vi "OCR Player Money.vi"(7 "error in":errorcluster) -> (17 "String (Player10 Money)":string, 18 "String (Player 9 Money)":string, 19 "String (Player8 Money)":string, 20 "String (Player1 Money)":string, 21 "String (Player2 Money)":string, 22 "String (Player3 Money)":string, 23 "String (Player4 Money)":string, 24 "String (Player5 Money)":string, 25 "String (Player6 Money)":string, 26 "String (Player7 Money)":string, 27 "error out":errorcluster)   [LabVIEW 2015]
uses:
  <vilib>/vision/NI_Vision_Development_Module.lvlib
panel:
  out "Player Money":string[](array[string])
  in  "SS Path":path=path "c:/PokerSS/SS.png"
  out "Image Out":T1(plugin-control)
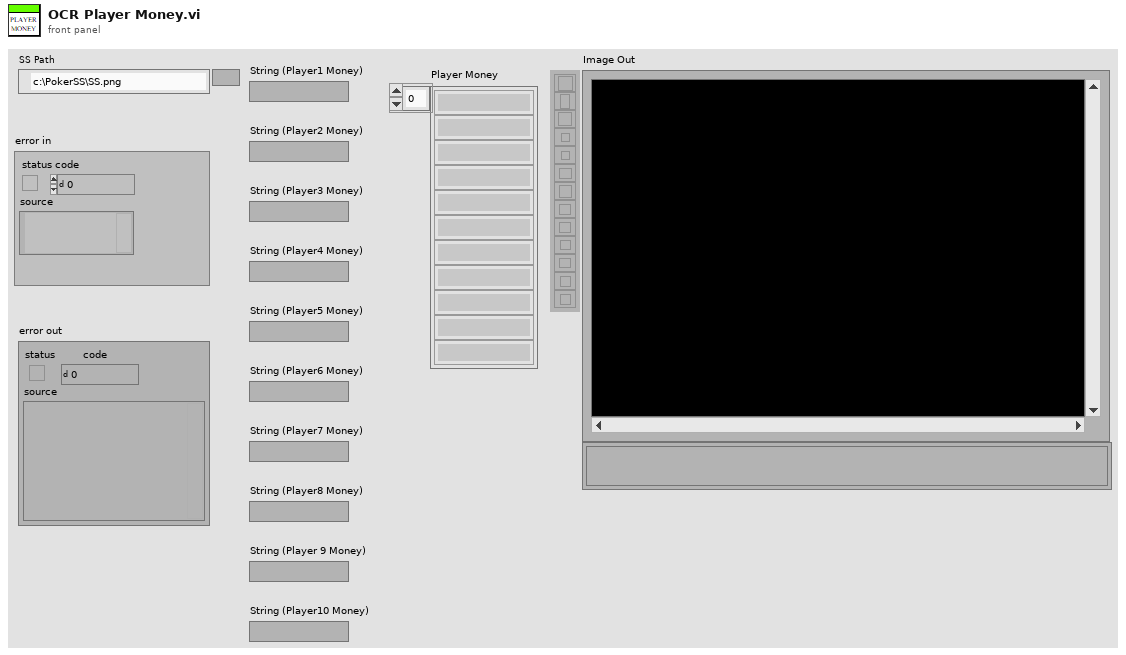
[diagram p1: front panel]
types:
  T1 = typedef "IMAQ Image.ctl" = refnum<image>
  T2 = cluster{"Threshold Data":cluster{"Method":enum16{"Fixed Range", "Uniform", "Linear", "Non Linear", "Local", "Color"}, "Looking for":u32, "Color Mode":u32, "Kernel Size":cluster{"Width":i32, "Height":i32}, "Ranges":cluster{"Min":i32, "Max":i32}[]}, "Reject Border":bool, "Number Of Erosions":i32, "Size & Spacing":cluster{"Segment Algorithm":u16, "Min Bounding Rect Width":i32, "Max Bounding Rect Width":i32, "Min Bounding Rect Height":i32, "Max Bounding Rect Height":i32, "Min Character Size":i32, "Max Character Size":i32, "Min Char Spacing":i32, "Max Horiz Element Spacing":i32, "Max Vert Element Spacing":i32, "Max Space Distance":i32}, "Read Options":cluster{"Read Strategy":i32, "Read Resolution":i32, "Scale Dependant":bool, "Aspect Ratio":i32, "Acceptance Level":i32, "Substitution Character":string, "MultiLine":bool}, "Valid Characters":cluster{"Pre-defined characters":i32, "User-defined characters":string}[], "Use Text Pattern":bool, "Orientation":u32, "# Lines Expected":u32, "Number of Blocks":i32}
  T3 = cluster{"Global Rectangle":i32[], "Contours":cluster{"ID":enum32{"External", "Internal"}, "Type":u32, "Coordinates":i32[]}[]}
  T4 = typedef "Image Type" = u32
  T5 = typedef "IMAQ OCR Session.ctl" = refnum<k1>
diagram:
  (unwired) path "C:/Users/Bob Dabalina/Documents/Labview/OCR Practice/Views Numbers.abc" ("File Path")
  w26 = u32 0 items=["Grayscale", "Binary", "Gradient", "Rainbow", "Temperature", "User Defined", "Binary 16 Bit", "Gradient 16 Bit", "Rainbow 16 Bit", "Temperature 16 Bit", "User Defined 16 Bit"] ("Palette Type")
  w35 = T2 {"Threshold Data"={"Method"=enum."Uniform", "Looking for"=1, "Color Mode"=0, "Kernel Size"={"Width"=32, "Height"=32}, "Ranges"=[{"Min"=1, "Max"=255}]}, "Reject Border"=TRUE, "Number Of Erosions"=0, "Size & Spacing"={"Segment Algorithm"=0, "Min Bounding Rect Width"=2, "Max Bounding Rect Width"=8, "Min Bounding Rect Height"=2, "Max Bounding Rect Height"=65536, "Min Character Size"=4, "Max Character Size"=5555, "Min Char Spacing"=1, "Max Horiz Element Spacing"=1, "Max Vert Element Spacing"=0, "Max Space Distance"=65536}, "Read Options"={"Read Strategy"=1, "Read Resolution"=2, "Scale Dependant"=FALSE, "Aspect Ratio"=400, "Acceptance Level"=700, "Substitution Character"="?", "MultiLine"=FALSE}, "Valid Characters"=[], "Use Text Pattern"=FALSE, "Orientation"=0, "# Lines Expected"=0, "Number of Blocks"=4}  # Parameters
  w36 = T3 {"Global Rectangle"=[720, 494, 833, 510], "Contours"=[{"ID"=enum."External", "Type"=3, "Coordinates"=[720, 494, 833, 510]}]}  # ROI Descriptor
  w44 = T2 {"Threshold Data"={"Method"=enum."Uniform", "Looking for"=1, "Color Mode"=0, "Kernel Size"={"Width"=32, "Height"=32}, "Ranges"=[{"Min"=1, "Max"=255}]}, "Reject Border"=TRUE, "Number Of Erosions"=0, "Size & Spacing"={"Segment Algorithm"=0, "Min Bounding Rect Width"=2, "Max Bounding Rect Width"=8, "Min Bounding Rect Height"=2, "Max Bounding Rect Height"=65536, "Min Character Size"=4, "Max Character Size"=5555, "Min Char Spacing"=1, "Max Horiz Element Spacing"=1, "Max Vert Element Spacing"=0, "Max Space Distance"=65536}, "Read Options"={"Read Strategy"=1, "Read Resolution"=2, "Scale Dependant"=FALSE, "Aspect Ratio"=400, "Acceptance Level"=700, "Substitution Character"="?", "MultiLine"=FALSE}, "Valid Characters"=[], "Use Text Pattern"=FALSE, "Orientation"=0, "# Lines Expected"=0, "Number of Blocks"=4}  # Parameters
  w45 = T3 {"Global Rectangle"=[523, 533, 645, 550], "Contours"=[{"ID"=enum."External", "Type"=3, "Coordinates"=[523, 533, 645, 550]}]}  # ROI Descriptor
  w53 = T2 {"Threshold Data"={"Method"=enum."Uniform", "Looking for"=1, "Color Mode"=0, "Kernel Size"={"Width"=32, "Height"=32}, "Ranges"=[{"Min"=1, "Max"=255}]}, "Reject Border"=TRUE, "Number Of Erosions"=0, "Size & Spacing"={"Segment Algorithm"=0, "Min Bounding Rect Width"=2, "Max Bounding Rect Width"=8, "Min Bounding Rect Height"=2, "Max Bounding Rect Height"=65536, "Min Character Size"=4, "Max Character Size"=5555, "Min Char Spacing"=1, "Max Horiz Element Spacing"=1, "Max Vert Element Spacing"=0, "Max Space Distance"=65536}, "Read Options"={"Read Strategy"=1, "Read Resolution"=2, "Scale Dependant"=FALSE, "Aspect Ratio"=400, "Acceptance Level"=700, "Substitution Character"="?", "MultiLine"=FALSE}, "Valid Characters"=[], "Use Text Pattern"=FALSE, "Orientation"=0, "# Lines Expected"=0, "Number of Blocks"=4}  # Parameters
  w54 = T3 {"Global Rectangle"=[386, 689, 502, 706], "Contours"=[{"ID"=enum."External", "Type"=3, "Coordinates"=[386, 689, 502, 706]}]}  # ROI Descriptor
  w62 = T2 {"Threshold Data"={"Method"=enum."Uniform", "Looking for"=1, "Color Mode"=0, "Kernel Size"={"Width"=32, "Height"=32}, "Ranges"=[{"Min"=1, "Max"=255}]}, "Reject Border"=TRUE, "Number Of Erosions"=0, "Size & Spacing"={"Segment Algorithm"=0, "Min Bounding Rect Width"=2, "Max Bounding Rect Width"=8, "Min Bounding Rect Height"=2, "Max Bounding Rect Height"=65536, "Min Character Size"=4, "Max Character Size"=5555, "Min Char Spacing"=1, "Max Horiz Element Spacing"=1, "Max Vert Element Spacing"=0, "Max Space Distance"=65536}, "Read Options"={"Read Strategy"=1, "Read Resolution"=2, "Scale Dependant"=FALSE, "Aspect Ratio"=400, "Acceptance Level"=700, "Substitution Character"="?", "MultiLine"=FALSE}, "Valid Characters"=[], "Use Text Pattern"=FALSE, "Orientation"=0, "# Lines Expected"=0, "Number of Blocks"=4}  # Parameters
  w63 = T3 {"Global Rectangle"=[543, 836, 661, 852], "Contours"=[{"ID"=enum."External", "Type"=3, "Coordinates"=[543, 836, 661, 852]}]}  # ROI Descriptor
  w71 = T2 {"Threshold Data"={"Method"=enum."Uniform", "Looking for"=1, "Color Mode"=0, "Kernel Size"={"Width"=32, "Height"=32}, "Ranges"=[{"Min"=1, "Max"=255}]}, "Reject Border"=TRUE, "Number Of Erosions"=0, "Size & Spacing"={"Segment Algorithm"=0, "Min Bounding Rect Width"=2, "Max Bounding Rect Width"=8, "Min Bounding Rect Height"=2, "Max Bounding Rect Height"=65536, "Min Character Size"=4, "Max Character Size"=5555, "Min Char Spacing"=1, "Max Horiz Element Spacing"=1, "Max Vert Element Spacing"=0, "Max Space Distance"=65536}, "Read Options"={"Read Strategy"=1, "Read Resolution"=2, "Scale Dependant"=FALSE, "Aspect Ratio"=400, "Acceptance Level"=700, "Substitution Character"="?", "MultiLine"=FALSE}, "Valid Characters"=[], "Use Text Pattern"=FALSE, "Orientation"=0, "# Lines Expected"=0, "Number of Blocks"=4}  # Parameters
  w72 = T3 {"Global Rectangle"=[757, 870, 877, 885], "Contours"=[{"ID"=enum."External", "Type"=3, "Coordinates"=[757, 870, 877, 885]}]}  # ROI Descriptor
  w80 = T2 {"Threshold Data"={"Method"=enum."Uniform", "Looking for"=1, "Color Mode"=0, "Kernel Size"={"Width"=32, "Height"=32}, "Ranges"=[{"Min"=1, "Max"=255}]}, "Reject Border"=TRUE, "Number Of Erosions"=0, "Size & Spacing"={"Segment Algorithm"=0, "Min Bounding Rect Width"=2, "Max Bounding Rect Width"=8, "Min Bounding Rect Height"=2, "Max Bounding Rect Height"=65536, "Min Character Size"=4, "Max Character Size"=5555, "Min Char Spacing"=1, "Max Horiz Element Spacing"=1, "Max Vert Element Spacing"=0, "Max Space Distance"=65536}, "Read Options"={"Read Strategy"=1, "Read Resolution"=2, "Scale Dependant"=FALSE, "Aspect Ratio"=400, "Acceptance Level"=700, "Substitution Character"="?", "MultiLine"=FALSE}, "Valid Characters"=[], "Use Text Pattern"=FALSE, "Orientation"=0, "# Lines Expected"=0, "Number of Blocks"=4}  # Parameters
  w81 = T3 {"Global Rectangle"=[1029, 868, 1143, 884], "Contours"=[{"ID"=enum."External", "Type"=3, "Coordinates"=[1029, 868, 1143, 884]}]}  # ROI Descriptor
  w89 = T2 {"Threshold Data"={"Method"=enum."Uniform", "Looking for"=1, "Color Mode"=0, "Kernel Size"={"Width"=32, "Height"=32}, "Ranges"=[{"Min"=1, "Max"=255}]}, "Reject Border"=TRUE, "Number Of Erosions"=0, "Size & Spacing"={"Segment Algorithm"=0, "Min Bounding Rect Width"=2, "Max Bounding Rect Width"=8, "Min Bounding Rect Height"=2, "Max Bounding Rect Height"=65536, "Min Character Size"=4, "Max Character Size"=5555, "Min Char Spacing"=1, "Max Horiz Element Spacing"=1, "Max Vert Element Spacing"=0, "Max Space Distance"=65536}, "Read Options"={"Read Strategy"=1, "Read Resolution"=2, "Scale Dependant"=FALSE, "Aspect Ratio"=400, "Acceptance Level"=700, "Substitution Character"="?", "MultiLine"=FALSE}, "Valid Characters"=[], "Use Text Pattern"=FALSE, "Orientation"=0, "# Lines Expected"=0, "Number of Blocks"=4}  # Parameters
  w90 = T3 {"Global Rectangle"=[1264, 838, 1374, 853], "Contours"=[{"ID"=enum."External", "Type"=3, "Coordinates"=[1264, 838, 1374, 853]}]}  # ROI Descriptor
  w98 = T2 {"Threshold Data"={"Method"=enum."Uniform", "Looking for"=1, "Color Mode"=0, "Kernel Size"={"Width"=32, "Height"=32}, "Ranges"=[{"Min"=1, "Max"=255}]}, "Reject Border"=TRUE, "Number Of Erosions"=0, "Size & Spacing"={"Segment Algorithm"=0, "Min Bounding Rect Width"=2, "Max Bounding Rect Width"=8, "Min Bounding Rect Height"=2, "Max Bounding Rect Height"=65536, "Min Character Size"=4, "Max Character Size"=5555, "Min Char Spacing"=1, "Max Horiz Element Spacing"=1, "Max Vert Element Spacing"=0, "Max Space Distance"=65536}, "Read Options"={"Read Strategy"=1, "Read Resolution"=2, "Scale Dependant"=FALSE, "Aspect Ratio"=400, "Acceptance Level"=700, "Substitution Character"="?", "MultiLine"=FALSE}, "Valid Characters"=[], "Use Text Pattern"=FALSE, "Orientation"=0, "# Lines Expected"=0, "Number of Blocks"=4}  # Parameters
  w99 = T3 {"Global Rectangle"=[1385, 697, 1502, 712], "Contours"=[{"ID"=enum."External", "Type"=3, "Coordinates"=[1385, 697, 1502, 712]}]}  # ROI Descriptor
  w107 = T2 {"Threshold Data"={"Method"=enum."Uniform", "Looking for"=1, "Color Mode"=0, "Kernel Size"={"Width"=32, "Height"=32}, "Ranges"=[{"Min"=1, "Max"=255}]}, "Reject Border"=TRUE, "Number Of Erosions"=0, "Size & Spacing"={"Segment Algorithm"=0, "Min Bounding Rect Width"=2, "Max Bounding Rect Width"=8, "Min Bounding Rect Height"=2, "Max Bounding Rect Height"=65536, "Min Character Size"=4, "Max Character Size"=5555, "Min Char Spacing"=1, "Max Horiz Element Spacing"=1, "Max Vert Element Spacing"=0, "Max Space Distance"=65536}, "Read Options"={"Read Strategy"=1, "Read Resolution"=2, "Scale Dependant"=FALSE, "Aspect Ratio"=400, "Acceptance Level"=700, "Substitution Character"="?", "MultiLine"=FALSE}, "Valid Characters"=[], "Use Text Pattern"=FALSE, "Orientation"=0, "# Lines Expected"=0, "Number of Blocks"=4}  # Parameters
  w108 = T3 {"Global Rectangle"=[1068, 495, 1179, 512], "Contours"=[{"ID"=enum."External", "Type"=3, "Coordinates"=[1068, 495, 1179, 512]}]}  # ROI Descriptor
  w116 = T2 {"Threshold Data"={"Method"=enum."Uniform", "Looking for"=1, "Color Mode"=0, "Kernel Size"={"Width"=32, "Height"=32}, "Ranges"=[{"Min"=1, "Max"=255}]}, "Reject Border"=TRUE, "Number Of Erosions"=0, "Size & Spacing"={"Segment Algorithm"=0, "Min Bounding Rect Width"=2, "Max Bounding Rect Width"=8, "Min Bounding Rect Height"=2, "Max Bounding Rect Height"=65536, "Min Character Size"=4, "Max Character Size"=5555, "Min Char Spacing"=1, "Max Horiz Element Spacing"=1, "Max Vert Element Spacing"=0, "Max Space Distance"=65536}, "Read Options"={"Read Strategy"=1, "Read Resolution"=2, "Scale Dependant"=FALSE, "Aspect Ratio"=400, "Acceptance Level"=700, "Substitution Character"="?", "MultiLine"=FALSE}, "Valid Characters"=[], "Use Text Pattern"=FALSE, "Orientation"=0, "# Lines Expected"=0, "Number of Blocks"=4}  # Parameters
  w117 = T3 {"Global Rectangle"=[1068, 495, 1179, 512], "Contours"=[{"ID"=enum."External", "Type"=3, "Coordinates"=[1068, 495, 1179, 512]}]}  # ROI Descriptor
  w120 = 1 items=["Red", "Green", "Blue", "Hue", "Saturation", "Luminance", "Value", "Intensity"] ("Color Plane")
  w121 = T4 4 items=["Grayscale (U8)", "Grayscale (I16)", "Grayscale (SGL)", "Complex (CSG)", "RGB (U32)", "HSL (U32)", "RGB (U64)", "Grayscale (U16)"] ("Image Type")
  # "Create player money array"
  n1 = Call Chain() -> (call chain=w123:string[])
  n2 = Index Array(array=w123) -> (element=w122:string)  [unwired: 1 in]
  n3 = call "IMAQ Create"("Image Name"=w122, "Image Type"=w121, "error in (no error)"="error in") -> ("New Image"=w126:T1, "error out"=w125:errorcluster)  [unwired: 1 in, 1 out]
  n4 = call "IMAQ ReadFile"("File Path"="SS Path", "error in (no error)"=w125, "Image"=w126) -> ("error out"=w127:errorcluster, "Image Out"=w119:T1)  [unwired: 2 in, 5 out]
  n5 = call "IMAQ ExtractSingleColorPlane"("Color Plane"=w120, "error in (no error)"=w127, "Image Src"=w119) -> ("error out"=w118:errorcluster, "Image Dst Out"=w27:T1)  [unwired: 1 in, 6 out]
  "Image Out" <- w27
  n6 = while "Create an OCR session and read the character set file.\nSet paramaters from Vision Assistant Step." {
    shift-right: [w132] -> w114
    shift-left: _ -> [w131]
    tunnel: w118 -> [w134]
    tunnel: w116 -> [w130]
    tunnel: path "C:/Users/Bob Dabalina/Documents/Labview/OCR Practice/Views Numbers.abc" ("File Path") -> [w129]
    tunnel: [w128] -> w115
    stop <- FALSE continue-if-true
    n7 = First Call?() -> (First Call?: T/F=w133:bool)
    n8 = case shown="True" w133 {
      tunnel: w129 -> [_ w141]
      tunnel: w134 -> [w136 w145]
      tunnel: [w137 w143] -> w132
      tunnel: [w136 w142] -> w128
      tunnel: w130 -> [_ w138]
      tunnel: w131 -> [w137 _]
      frame False {
      }
      frame True {
        w146 = 0 items=["Read All", "Read Character Set Only", "Read Properties Only"] ("Read Options")
        n9 = call <vilib>:"IVA Get Alternate Path.vi"("Path In"=w141) -> ("Path Out"=w140:path)  [unwired: 10 out]
        n10 = call "IMAQ OCR Create Session"("error in (no error)"=w145) -> ("error out"=w147:errorcluster, "IMAQ OCR Session"=w148:T5)  [unwired: 9 out]
        n11 = call "IMAQ OCR Read Character Set File"("File Path"=w140, "error in (no error)"=w147, "Read Options"=w146, "IMAQ OCR Session"=w148) -> ("error out"=w144:errorcluster, "IMAQ OCR Session (dup)"=w139:T5)  [unwired: 1 in, 5 out]
        n12 = call <vilib>:"IVA OCR - Set Parameters 2.vi"("error in (no error)"=w144, "Parameters"=w138, "IMAQ OCR Session"=w139) -> ("error out"=w142:errorcluster, "IMAQ OCR Session Out"=w143:T5)  [unwired: 7 in]
      }
    }
  }
  n13 = Unbundle By Name(w116) -> ("# Lines Expected"=w112:u32, "Orientation"=w113:u32)
  n14 = call "IMAQ OCR Read Text 4"("IMAQ OCR Session"=w114, "ROI Descriptor"=w117, "Image"=w27, "Number of Lines Requested"=w112, "error in (no error)"=w115, "Orientation"=w113) -> ("Read String"=w20:string, "error out"=w111:errorcluster)  [unwired: 8 out]
  "String (Player1 Money)" <- w20
  n15 = call <vilib>:"IVA Clear Coordsys Errors.vi"("error in (no error)"=w111) -> ("error out"=w110:errorcluster)  [unwired: 10 in]
  n16 = Initialize Array("") -> (w22:string[])  [unwired: 1 in]
  n17 = Insert Into Array(array=w22, index=0, new element=w20) -> (w19:string[])
  n18 = while "Create an OCR session and read the character set file.\nSet paramaters from Vision Assistant Step." {
    shift-right: [w153] -> w105
    shift-left: _ -> [w152]
    tunnel: w110 -> [w155]
    tunnel: w107 -> [w151]
    tunnel: path "C:/Users/Bob Dabalina/Documents/Labview/OCR Practice/Views Numbers.abc" ("File Path") -> [w150]
    tunnel: [w149] -> w106
    stop <- FALSE continue-if-true
    n19 = First Call?() -> (First Call?: T/F=w154:bool)
    n20 = case shown="True" w154 {
      tunnel: w150 -> [_ w162]
      tunnel: w155 -> [w157 w166]
      tunnel: [w158 w164] -> w153
      tunnel: [w157 w163] -> w149
      tunnel: w151 -> [_ w159]
      tunnel: w152 -> [w158 _]
      frame False {
      }
      frame True {
        w167 = 0 items=["Read All", "Read Character Set Only", "Read Properties Only"] ("Read Options")
        n21 = call <vilib>:"IVA Get Alternate Path.vi"("Path In"=w162) -> ("Path Out"=w161:path)  [unwired: 10 out]
        n22 = call "IMAQ OCR Create Session"("error in (no error)"=w166) -> ("error out"=w168:errorcluster, "IMAQ OCR Session"=w169:T5)  [unwired: 9 out]
        n23 = call "IMAQ OCR Read Character Set File"("File Path"=w161, "error in (no error)"=w168, "Read Options"=w167, "IMAQ OCR Session"=w169) -> ("error out"=w165:errorcluster, "IMAQ OCR Session (dup)"=w160:T5)  [unwired: 1 in, 5 out]
        n24 = call <vilib>:"IVA OCR - Set Parameters 2.vi"("error in (no error)"=w165, "Parameters"=w159, "IMAQ OCR Session"=w160) -> ("error out"=w163:errorcluster, "IMAQ OCR Session Out"=w164:T5)  [unwired: 7 in]
      }
    }
  }
  n25 = Unbundle By Name(w107) -> ("# Lines Expected"=w103:u32, "Orientation"=w104:u32)
  n26 = call "IMAQ OCR Read Text 4"("IMAQ OCR Session"=w105, "ROI Descriptor"=w108, "Image"=w27, "Number of Lines Requested"=w103, "error in (no error)"=w106, "Orientation"=w104) -> ("Read String"=w18:string, "error out"=w102:errorcluster)  [unwired: 8 out]
  "String (Player2 Money)" <- w18
  n27 = call <vilib>:"IVA Clear Coordsys Errors.vi"("error in (no error)"=w102) -> ("error out"=w101:errorcluster)  [unwired: 10 in]
  n28 = Build Array (concatenate)(w19, w18) -> (w17:string[])
  n29 = while "Create an OCR session and read the character set file.\nSet paramaters from Vision Assistant Step." {
    shift-right: [w174] -> w96
    shift-left: _ -> [w173]
    tunnel: w101 -> [w176]
    tunnel: w98 -> [w172]
    tunnel: path "C:/Users/Bob Dabalina/Documents/Labview/OCR Practice/Views Numbers.abc" ("File Path") -> [w171]
    tunnel: [w170] -> w97
    stop <- FALSE continue-if-true
    n30 = First Call?() -> (First Call?: T/F=w175:bool)
    n31 = case shown="True" w175 {
      tunnel: w171 -> [_ w183]
      tunnel: w176 -> [w178 w187]
      tunnel: [w179 w185] -> w174
      tunnel: [w178 w184] -> w170
      tunnel: w172 -> [_ w180]
      tunnel: w173 -> [w179 _]
      frame False {
      }
      frame True {
        w188 = 0 items=["Read All", "Read Character Set Only", "Read Properties Only"] ("Read Options")
        n32 = call <vilib>:"IVA Get Alternate Path.vi"("Path In"=w183) -> ("Path Out"=w182:path)  [unwired: 10 out]
        n33 = call "IMAQ OCR Create Session"("error in (no error)"=w187) -> ("error out"=w189:errorcluster, "IMAQ OCR Session"=w190:T5)  [unwired: 9 out]
        n34 = call "IMAQ OCR Read Character Set File"("File Path"=w182, "error in (no error)"=w189, "Read Options"=w188, "IMAQ OCR Session"=w190) -> ("error out"=w186:errorcluster, "IMAQ OCR Session (dup)"=w181:T5)  [unwired: 1 in, 5 out]
        n35 = call <vilib>:"IVA OCR - Set Parameters 2.vi"("error in (no error)"=w186, "Parameters"=w180, "IMAQ OCR Session"=w181) -> ("error out"=w184:errorcluster, "IMAQ OCR Session Out"=w185:T5)  [unwired: 7 in]
      }
    }
  }
  n36 = Unbundle By Name(w98) -> ("# Lines Expected"=w94:u32, "Orientation"=w95:u32)
  n37 = call "IMAQ OCR Read Text 4"("IMAQ OCR Session"=w96, "ROI Descriptor"=w99, "Image"=w27, "Number of Lines Requested"=w94, "error in (no error)"=w97, "Orientation"=w95) -> ("Read String"=w16:string, "error out"=w93:errorcluster)  [unwired: 8 out]
  "String (Player3 Money)" <- w16
  n38 = call <vilib>:"IVA Clear Coordsys Errors.vi"("error in (no error)"=w93) -> ("error out"=w92:errorcluster)  [unwired: 10 in]
  n39 = Build Array (concatenate)(w17, w16) -> (w15:string[])
  n40 = while "Create an OCR session and read the character set file.\nSet paramaters from Vision Assistant Step." {
    shift-right: [w195] -> w87
    shift-left: _ -> [w194]
    tunnel: w92 -> [w197]
    tunnel: w89 -> [w193]
    tunnel: path "C:/Users/Bob Dabalina/Documents/Labview/OCR Practice/Views Numbers.abc" ("File Path") -> [w192]
    tunnel: [w191] -> w88
    stop <- FALSE continue-if-true
    n41 = First Call?() -> (First Call?: T/F=w196:bool)
    n42 = case shown="True" w196 {
      tunnel: w192 -> [_ w204]
      tunnel: w197 -> [w199 w208]
      tunnel: [w200 w206] -> w195
      tunnel: [w199 w205] -> w191
      tunnel: w193 -> [_ w201]
      tunnel: w194 -> [w200 _]
      frame False {
      }
      frame True {
        w209 = 0 items=["Read All", "Read Character Set Only", "Read Properties Only"] ("Read Options")
        n43 = call <vilib>:"IVA Get Alternate Path.vi"("Path In"=w204) -> ("Path Out"=w203:path)  [unwired: 10 out]
        n44 = call "IMAQ OCR Create Session"("error in (no error)"=w208) -> ("error out"=w210:errorcluster, "IMAQ OCR Session"=w211:T5)  [unwired: 9 out]
        n45 = call "IMAQ OCR Read Character Set File"("File Path"=w203, "error in (no error)"=w210, "Read Options"=w209, "IMAQ OCR Session"=w211) -> ("error out"=w207:errorcluster, "IMAQ OCR Session (dup)"=w202:T5)  [unwired: 1 in, 5 out]
        n46 = call <vilib>:"IVA OCR - Set Parameters 2.vi"("error in (no error)"=w207, "Parameters"=w201, "IMAQ OCR Session"=w202) -> ("error out"=w205:errorcluster, "IMAQ OCR Session Out"=w206:T5)  [unwired: 7 in]
      }
    }
  }
  n47 = Unbundle By Name(w89) -> ("# Lines Expected"=w85:u32, "Orientation"=w86:u32)
  n48 = call "IMAQ OCR Read Text 4"("IMAQ OCR Session"=w87, "ROI Descriptor"=w90, "Image"=w27, "Number of Lines Requested"=w85, "error in (no error)"=w88, "Orientation"=w86) -> ("Read String"=w14:string, "error out"=w84:errorcluster)  [unwired: 8 out]
  "String (Player4 Money)" <- w14
  n49 = call <vilib>:"IVA Clear Coordsys Errors.vi"("error in (no error)"=w84) -> ("error out"=w83:errorcluster)  [unwired: 10 in]
  n50 = Build Array (concatenate)(w15, w14) -> (w13:string[])
  n51 = while "Create an OCR session and read the character set file.\nSet paramaters from Vision Assistant Step." {
    shift-right: [w216] -> w78
    shift-left: _ -> [w215]
    tunnel: w83 -> [w218]
    tunnel: w80 -> [w214]
    tunnel: path "C:/Users/Bob Dabalina/Documents/Labview/OCR Practice/Views Numbers.abc" ("File Path") -> [w213]
    tunnel: [w212] -> w79
    stop <- FALSE continue-if-true
    n52 = First Call?() -> (First Call?: T/F=w217:bool)
    n53 = case shown="True" w217 {
      tunnel: w213 -> [_ w225]
      tunnel: w218 -> [w220 w229]
      tunnel: [w221 w227] -> w216
      tunnel: [w220 w226] -> w212
      tunnel: w214 -> [_ w222]
      tunnel: w215 -> [w221 _]
      frame False {
      }
      frame True {
        w230 = 0 items=["Read All", "Read Character Set Only", "Read Properties Only"] ("Read Options")
        n54 = call <vilib>:"IVA Get Alternate Path.vi"("Path In"=w225) -> ("Path Out"=w224:path)  [unwired: 10 out]
        n55 = call "IMAQ OCR Create Session"("error in (no error)"=w229) -> ("error out"=w231:errorcluster, "IMAQ OCR Session"=w232:T5)  [unwired: 9 out]
        n56 = call "IMAQ OCR Read Character Set File"("File Path"=w224, "error in (no error)"=w231, "Read Options"=w230, "IMAQ OCR Session"=w232) -> ("error out"=w228:errorcluster, "IMAQ OCR Session (dup)"=w223:T5)  [unwired: 1 in, 5 out]
        n57 = call <vilib>:"IVA OCR - Set Parameters 2.vi"("error in (no error)"=w228, "Parameters"=w222, "IMAQ OCR Session"=w223) -> ("error out"=w226:errorcluster, "IMAQ OCR Session Out"=w227:T5)  [unwired: 7 in]
      }
    }
  }
  n58 = Unbundle By Name(w80) -> ("# Lines Expected"=w76:u32, "Orientation"=w77:u32)
  n59 = call "IMAQ OCR Read Text 4"("IMAQ OCR Session"=w78, "ROI Descriptor"=w81, "Image"=w27, "Number of Lines Requested"=w76, "error in (no error)"=w79, "Orientation"=w77) -> ("Read String"=w12:string, "error out"=w75:errorcluster)  [unwired: 8 out]
  "String (Player5 Money)" <- w12
  n60 = call <vilib>:"IVA Clear Coordsys Errors.vi"("error in (no error)"=w75) -> ("error out"=w74:errorcluster)  [unwired: 10 in]
  n61 = Build Array (concatenate)(w13, w12) -> (w11:string[])
  n62 = while "Create an OCR session and read the character set file.\nSet paramaters from Vision Assistant Step." {
    shift-right: [w237] -> w69
    shift-left: _ -> [w236]
    tunnel: w74 -> [w239]
    tunnel: w71 -> [w235]
    tunnel: path "C:/Users/Bob Dabalina/Documents/Labview/OCR Practice/Views Numbers.abc" ("File Path") -> [w234]
    tunnel: [w233] -> w70
    stop <- FALSE continue-if-true
    n63 = First Call?() -> (First Call?: T/F=w238:bool)
    n64 = case shown="True" w238 {
      tunnel: w234 -> [_ w246]
      tunnel: w239 -> [w241 w250]
      tunnel: [w242 w248] -> w237
      tunnel: [w241 w247] -> w233
      tunnel: w235 -> [_ w243]
      tunnel: w236 -> [w242 _]
      frame False {
      }
      frame True {
        w251 = 0 items=["Read All", "Read Character Set Only", "Read Properties Only"] ("Read Options")
        n65 = call <vilib>:"IVA Get Alternate Path.vi"("Path In"=w246) -> ("Path Out"=w245:path)  [unwired: 10 out]
        n66 = call "IMAQ OCR Create Session"("error in (no error)"=w250) -> ("error out"=w252:errorcluster, "IMAQ OCR Session"=w253:T5)  [unwired: 9 out]
        n67 = call "IMAQ OCR Read Character Set File"("File Path"=w245, "error in (no error)"=w252, "Read Options"=w251, "IMAQ OCR Session"=w253) -> ("error out"=w249:errorcluster, "IMAQ OCR Session (dup)"=w244:T5)  [unwired: 1 in, 5 out]
        n68 = call <vilib>:"IVA OCR - Set Parameters 2.vi"("error in (no error)"=w249, "Parameters"=w243, "IMAQ OCR Session"=w244) -> ("error out"=w247:errorcluster, "IMAQ OCR Session Out"=w248:T5)  [unwired: 7 in]
      }
    }
  }
  n69 = Unbundle By Name(w71) -> ("# Lines Expected"=w67:u32, "Orientation"=w68:u32)
  n70 = call "IMAQ OCR Read Text 4"("IMAQ OCR Session"=w69, "ROI Descriptor"=w72, "Image"=w27, "Number of Lines Requested"=w67, "error in (no error)"=w70, "Orientation"=w68) -> ("Read String"=w10:string, "error out"=w66:errorcluster)  [unwired: 8 out]
  "String (Player6 Money)" <- w10
  n71 = call <vilib>:"IVA Clear Coordsys Errors.vi"("error in (no error)"=w66) -> ("error out"=w65:errorcluster)  [unwired: 10 in]
  n72 = Build Array (concatenate)(w11, w10) -> (w9:string[])
  n73 = while "Create an OCR session and read the character set file.\nSet paramaters from Vision Assistant Step." {
    shift-right: [w258] -> w60
    shift-left: _ -> [w257]
    tunnel: w65 -> [w260]
    tunnel: w62 -> [w256]
    tunnel: path "C:/Users/Bob Dabalina/Documents/Labview/OCR Practice/Views Numbers.abc" ("File Path") -> [w255]
    tunnel: [w254] -> w61
    stop <- FALSE continue-if-true
    n74 = First Call?() -> (First Call?: T/F=w259:bool)
    n75 = case shown="True" w259 {
      tunnel: w255 -> [_ w267]
      tunnel: w260 -> [w262 w271]
      tunnel: [w263 w269] -> w258
      tunnel: [w262 w268] -> w254
      tunnel: w256 -> [_ w264]
      tunnel: w257 -> [w263 _]
      frame False {
      }
      frame True {
        w272 = 0 items=["Read All", "Read Character Set Only", "Read Properties Only"] ("Read Options")
        n76 = call <vilib>:"IVA Get Alternate Path.vi"("Path In"=w267) -> ("Path Out"=w266:path)  [unwired: 10 out]
        n77 = call "IMAQ OCR Create Session"("error in (no error)"=w271) -> ("error out"=w273:errorcluster, "IMAQ OCR Session"=w274:T5)  [unwired: 9 out]
        n78 = call "IMAQ OCR Read Character Set File"("File Path"=w266, "error in (no error)"=w273, "Read Options"=w272, "IMAQ OCR Session"=w274) -> ("error out"=w270:errorcluster, "IMAQ OCR Session (dup)"=w265:T5)  [unwired: 1 in, 5 out]
        n79 = call <vilib>:"IVA OCR - Set Parameters 2.vi"("error in (no error)"=w270, "Parameters"=w264, "IMAQ OCR Session"=w265) -> ("error out"=w268:errorcluster, "IMAQ OCR Session Out"=w269:T5)  [unwired: 7 in]
      }
    }
  }
  n80 = Unbundle By Name(w62) -> ("# Lines Expected"=w58:u32, "Orientation"=w59:u32)
  n81 = call "IMAQ OCR Read Text 4"("IMAQ OCR Session"=w60, "ROI Descriptor"=w63, "Image"=w27, "Number of Lines Requested"=w58, "error in (no error)"=w61, "Orientation"=w59) -> ("Read String"=w8:string, "error out"=w57:errorcluster)  [unwired: 8 out]
  "String (Player7 Money)" <- w8
  n82 = call <vilib>:"IVA Clear Coordsys Errors.vi"("error in (no error)"=w57) -> ("error out"=w56:errorcluster)  [unwired: 10 in]
  n83 = Build Array (concatenate)(w9, w8) -> (w7:string[])
  n84 = while "Create an OCR session and read the character set file.\nSet paramaters from Vision Assistant Step." {
    shift-right: [w279] -> w51
    shift-left: _ -> [w278]
    tunnel: w56 -> [w281]
    tunnel: w53 -> [w277]
    tunnel: path "C:/Users/Bob Dabalina/Documents/Labview/OCR Practice/Views Numbers.abc" ("File Path") -> [w276]
    tunnel: [w275] -> w52
    stop <- FALSE continue-if-true
    n85 = First Call?() -> (First Call?: T/F=w280:bool)
    n86 = case shown="True" w280 {
      tunnel: w276 -> [_ w288]
      tunnel: w281 -> [w283 w292]
      tunnel: [w284 w290] -> w279
      tunnel: [w283 w289] -> w275
      tunnel: w277 -> [_ w285]
      tunnel: w278 -> [w284 _]
      frame False {
      }
      frame True {
        w293 = 0 items=["Read All", "Read Character Set Only", "Read Properties Only"] ("Read Options")
        n87 = call <vilib>:"IVA Get Alternate Path.vi"("Path In"=w288) -> ("Path Out"=w287:path)  [unwired: 10 out]
        n88 = call "IMAQ OCR Create Session"("error in (no error)"=w292) -> ("error out"=w294:errorcluster, "IMAQ OCR Session"=w295:T5)  [unwired: 9 out]
        n89 = call "IMAQ OCR Read Character Set File"("File Path"=w287, "error in (no error)"=w294, "Read Options"=w293, "IMAQ OCR Session"=w295) -> ("error out"=w291:errorcluster, "IMAQ OCR Session (dup)"=w286:T5)  [unwired: 1 in, 5 out]
        n90 = call <vilib>:"IVA OCR - Set Parameters 2.vi"("error in (no error)"=w291, "Parameters"=w285, "IMAQ OCR Session"=w286) -> ("error out"=w289:errorcluster, "IMAQ OCR Session Out"=w290:T5)  [unwired: 7 in]
      }
    }
  }
  n91 = Unbundle By Name(w53) -> ("# Lines Expected"=w49:u32, "Orientation"=w50:u32)
  n92 = call "IMAQ OCR Read Text 4"("IMAQ OCR Session"=w51, "ROI Descriptor"=w54, "Image"=w27, "Number of Lines Requested"=w49, "error in (no error)"=w52, "Orientation"=w50) -> ("Read String"=w6:string, "error out"=w48:errorcluster)  [unwired: 8 out]
  "String (Player8 Money)" <- w6
  n93 = call <vilib>:"IVA Clear Coordsys Errors.vi"("error in (no error)"=w48) -> ("error out"=w47:errorcluster)  [unwired: 10 in]
  n94 = Build Array (concatenate)(w7, w6) -> (w5:string[])
  n95 = while "Create an OCR session and read the character set file.\nSet paramaters from Vision Assistant Step." {
    shift-right: [w300] -> w42
    shift-left: _ -> [w299]
    tunnel: w47 -> [w302]
    tunnel: w44 -> [w298]
    tunnel: path "C:/Users/Bob Dabalina/Documents/Labview/OCR Practice/Views Numbers.abc" ("File Path") -> [w297]
    tunnel: [w296] -> w43
    stop <- FALSE continue-if-true
    n96 = First Call?() -> (First Call?: T/F=w301:bool)
    n97 = case shown="True" w301 {
      tunnel: w297 -> [_ w309]
      tunnel: w302 -> [w304 w313]
      tunnel: [w305 w311] -> w300
      tunnel: [w304 w310] -> w296
      tunnel: w298 -> [_ w306]
      tunnel: w299 -> [w305 _]
      frame False {
      }
      frame True {
        w314 = 0 items=["Read All", "Read Character Set Only", "Read Properties Only"] ("Read Options")
        n98 = call <vilib>:"IVA Get Alternate Path.vi"("Path In"=w309) -> ("Path Out"=w308:path)  [unwired: 10 out]
        n99 = call "IMAQ OCR Create Session"("error in (no error)"=w313) -> ("error out"=w315:errorcluster, "IMAQ OCR Session"=w316:T5)  [unwired: 9 out]
        n100 = call "IMAQ OCR Read Character Set File"("File Path"=w308, "error in (no error)"=w315, "Read Options"=w314, "IMAQ OCR Session"=w316) -> ("error out"=w312:errorcluster, "IMAQ OCR Session (dup)"=w307:T5)  [unwired: 1 in, 5 out]
        n101 = call <vilib>:"IVA OCR - Set Parameters 2.vi"("error in (no error)"=w312, "Parameters"=w306, "IMAQ OCR Session"=w307) -> ("error out"=w310:errorcluster, "IMAQ OCR Session Out"=w311:T5)  [unwired: 7 in]
      }
    }
  }
  n102 = Unbundle By Name(w44) -> ("# Lines Expected"=w40:u32, "Orientation"=w41:u32)
  n103 = call "IMAQ OCR Read Text 4"("IMAQ OCR Session"=w42, "ROI Descriptor"=w45, "Image"=w27, "Number of Lines Requested"=w40, "error in (no error)"=w43, "Orientation"=w41) -> ("Read String"=w4:string, "error out"=w39:errorcluster)  [unwired: 8 out]
  "String (Player 9 Money)" <- w4
  n104 = call <vilib>:"IVA Clear Coordsys Errors.vi"("error in (no error)"=w39) -> ("error out"=w38:errorcluster)  [unwired: 10 in]
  n105 = Build Array (concatenate)(w5, w4) -> (w3:string[])
  n106 = while "Create an OCR session and read the character set file.\nSet paramaters from Vision Assistant Step." {
    shift-right: [w321] -> w33
    shift-left: _ -> [w320]
    tunnel: w38 -> [w323]
    tunnel: w35 -> [w319]
    tunnel: path "C:/Users/Bob Dabalina/Documents/Labview/OCR Practice/Views Numbers.abc" ("File Path") -> [w318]
    tunnel: [w317] -> w34
    stop <- FALSE continue-if-true
    n107 = First Call?() -> (First Call?: T/F=w322:bool)
    n108 = case shown="True" w322 {
      tunnel: w318 -> [_ w330]
      tunnel: w323 -> [w325 w334]
      tunnel: [w326 w332] -> w321
      tunnel: [w325 w331] -> w317
      tunnel: w319 -> [_ w327]
      tunnel: w320 -> [w326 _]
      frame False {
      }
      frame True {
        w335 = 0 items=["Read All", "Read Character Set Only", "Read Properties Only"] ("Read Options")
        n109 = call <vilib>:"IVA Get Alternate Path.vi"("Path In"=w330) -> ("Path Out"=w329:path)  [unwired: 10 out]
        n110 = call "IMAQ OCR Create Session"("error in (no error)"=w334) -> ("error out"=w336:errorcluster, "IMAQ OCR Session"=w337:T5)  [unwired: 9 out]
        n111 = call "IMAQ OCR Read Character Set File"("File Path"=w329, "error in (no error)"=w336, "Read Options"=w335, "IMAQ OCR Session"=w337) -> ("error out"=w333:errorcluster, "IMAQ OCR Session (dup)"=w328:T5)  [unwired: 1 in, 5 out]
        n112 = call <vilib>:"IVA OCR - Set Parameters 2.vi"("error in (no error)"=w333, "Parameters"=w327, "IMAQ OCR Session"=w328) -> ("error out"=w331:errorcluster, "IMAQ OCR Session Out"=w332:T5)  [unwired: 7 in]
      }
    }
  }
  n113 = Unbundle By Name(w35) -> ("# Lines Expected"=w31:u32, "Orientation"=w32:u32)
  n114 = call "IMAQ OCR Read Text 4"("IMAQ OCR Session"=w33, "ROI Descriptor"=w36, "Image"=w27, "Number of Lines Requested"=w31, "error in (no error)"=w34, "Orientation"=w32) -> ("Read String"=w2:string, "error out"=w30:errorcluster)  [unwired: 8 out]
  "String (Player10 Money)" <- w2
  n115 = call <vilib>:"IVA Clear Coordsys Errors.vi"("error in (no error)"=w30) -> ("error out"=w29:errorcluster)  [unwired: 10 in]
  n116 = property on="Image Out" class="ImageControl"(error in=w29, "Palette:Palette Type"=w26) -> (error out=→"error out":errorcluster)  [unwired: 1 in, 1 out]
  n117 = Build Array (concatenate)(w3, w2) -> (→"Player Money":string[])
